vi "Create Events.vi"(0 "Display State In":T2, 9 "Container State":T5, 11 "error in (no error)":errorcluster) -> (4 "Display State Out":T2, 8 "Events":T1, 15 "error out":errorcluster)   [LabVIEW 2015, in "FSM Editor.xctl"]
uses:
  FSM Editor.xctl
  <vilib>/_xctls/Container State.ctl
  State.vi
  Classes/FSM.Port/FSM.Port.lvclass
  <vilib>/Utility/miscctls.llb/LVPoint32TypeDef.ctl
  Drag Mode.ctl
  Events.ctl
  NodeAdded.ctl
  NodeSelected.ctl
  EdgeEventData.ctl
  <vilib>/_xctls/XControlSupport.lvlib
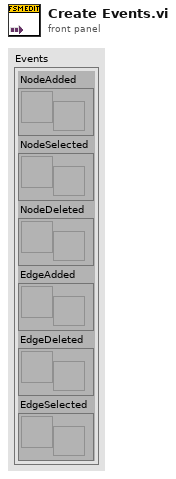
[diagram p1: front panel]
types:
  T1 = typedef "FSM Editor.xctl/Events.ctl" = cluster{"NodeAdded":refnum<user-event>, "NodeSelected":refnum<user-event>, "NodeDeleted":refnum<user-event>, "EdgeAdded":refnum<user-event>, "EdgeDeleted":refnum<user-event>, "EdgeSelected":refnum<user-event>}
  T2 = typedef "FSM Editor.xctl/State.vi" = cluster{"snap":bool, "default name":string, "dragStartPoint":T3, "dragMode":T4, "gridsize":dbl, "selectRect":cluster{"left":i16, "top":i16, "right":i16, "bottom":i16}, "events":string[], "cs+/cs-":bool, "insertEdgeAt":string, "insertingEdge":bool, "activePort":refnum<class "FSM.Port.lvclass">, "sourcePort":refnum<class "FSM.Port.lvclass">, "insertionEnd":cluster{"x":i16, "y":i16}, "insertEdgeSpec":string, "nodeIndex":i32, "Events":T1, "action":string}
  T3 = typedef "LVPoint32TypeDef.ctl" = cluster{"Horizontal":i32, "Vertical":i32}
  T4 = typedef "Drag Mode.ctl" = enum16{"Off", "NodePending", "Nodes", "Pan", "Select", "EdgeInsertion", "EdgePoint", "EdgeLabel"}
  T5 = typedef "XControlSupport.lvlib/Container State.ctl" = cluster{"Indicator?":bool, "Run Mode?":bool, " Refnum":refnum<vi>}
  T6 = typedef "FSM Editor.xctl/NodeSelected.ctl" = cluster{"Indices":i32[]}
  T7 = typedef "FSM Editor.xctl/EdgeEventData.ctl" = cluster{"Source":string, "Target":string, "Event":string, "Type":string}
  T8 = typedef "FSM Editor.xctl/NodeAdded.ctl" = cluster{"Name":string}
  T9 = cluster{"Event Data":refnum<user-event>, "Event Data":refnum<user-event>, "Event Data":refnum<user-event>, "Event Data":refnum<user-event>, "Event Data":refnum<user-event>, "Event Data":refnum<user-event>}
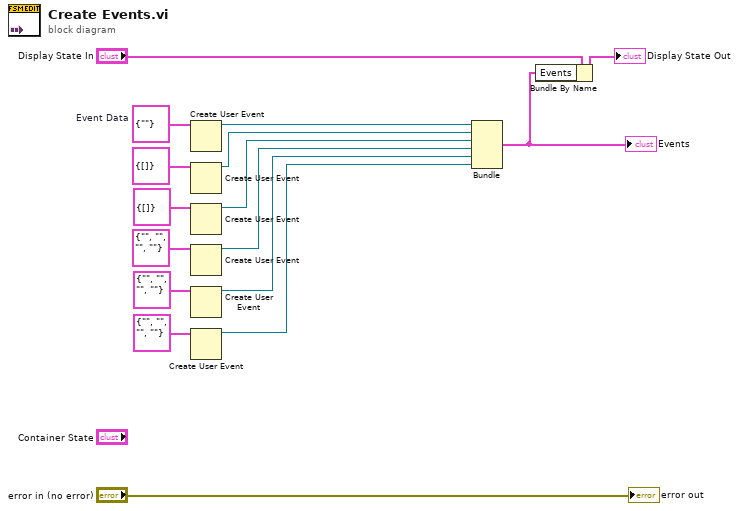
[diagram p0: block diagram]
diagram:
  w13 = T8 {"Name"=""}  # Event Data
  n1 = Create User Event(user event datatype=w13) -> (user event=w12:refnum<user-event>)  [unwired: 1 in, 1 out]
  n2 = Create User Event(user event datatype=T6 {"Indices"=[]} ("Event Data")) -> (user event=w9:refnum<user-event>)  [unwired: 1 in, 1 out]
  n3 = Create User Event(user event datatype=T6 {"Indices"=[]} ("Event Data")) -> (user event=w1:refnum<user-event>)  [unwired: 1 in, 1 out]
  n4 = Create User Event(user event datatype=T7 {"Source"="", "Target"="", "Event"="", "Type"=""} ("Event Data")) -> (user event=w7:refnum<user-event>)  [unwired: 1 in, 1 out]
  n5 = Create User Event(user event datatype=T7 {"Source"="", "Target"="", "Event"="", "Type"=""} ("Event Data")) -> (user event=w6:refnum<user-event>)  [unwired: 1 in, 1 out]
  n6 = Create User Event(user event datatype=T7 {"Source"="", "Target"="", "Event"="", "Type"=""} ("Event Data")) -> (user event=w4:refnum<user-event>)  [unwired: 1 in, 1 out]
  n7 = Bundle("Event Data"=w12, "Event Data"=w9, "Event Data"=w1, "Event Data"=w7, "Event Data"=w6, "Event Data"=w4) -> (w11:T9)  [unwired: 1 in]
  "Events" <- w11
  n8 = Bundle By Name(cluster="Display State In", "Events"=w11) -> (→"Display State Out":T2)
  "error out" <- "error in (no error)"
